vi "num_used_size.vi"(8 "error in (no error)":errorcluster, 11 "worksheet_Refnum":refnum<k7>) -> (0 "error out":errorcluster, 1 "Rows(0)":i32, 2 "Columns(0)":i32, 3 "worksheet_Refnum":refnum<k7>)   [LabVIEW 2015, in "Excel.lvclass"]
uses:
  Excel.lvclass
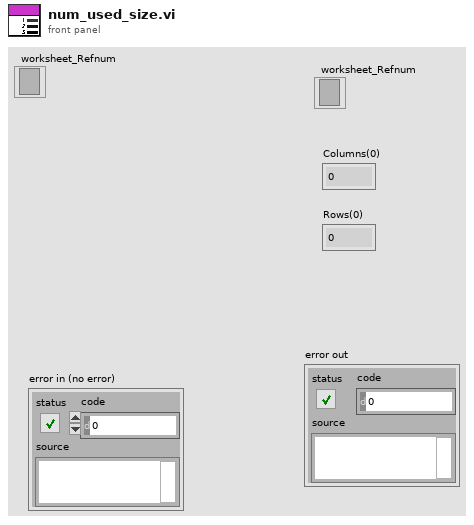
[diagram p1: front panel]
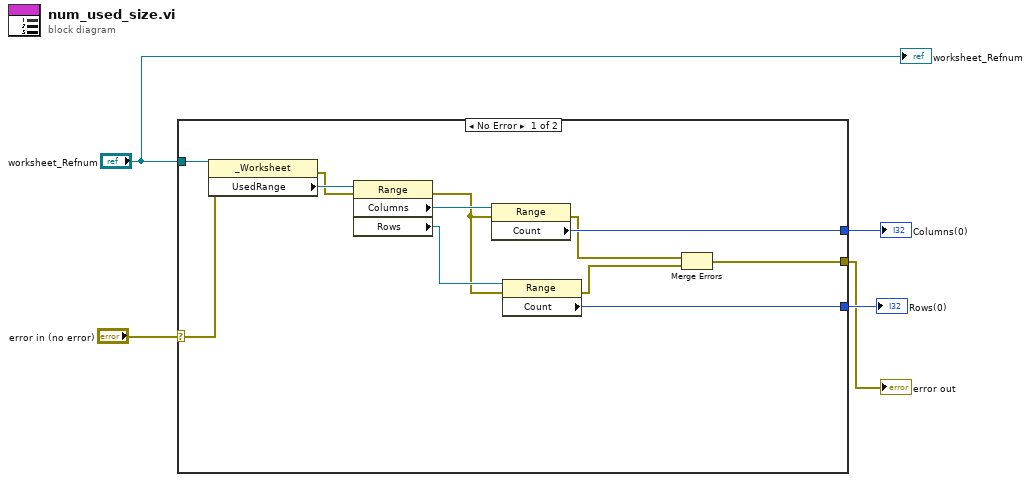
[diagram p0: block diagram]
diagram:
  n1 = case shown="No Error" "error in (no error)" {
    selector: "error in (no error)" -> [w12 w18]
    tunnel: [w16 _] -> w5
    tunnel: [w13 _] -> w4
    tunnel: [w7 w18] -> w2
    tunnel: "worksheet_Refnum" -> [w6 _]
    frame No Error {
      n2 = property class="_Worksheet"(reference=w6, error in=w12) -> (error out=w11:errorcluster, "UsedRange"=w14:refnum<k7>)  [unwired: 1 out]
      n3 = property class="Range"(reference=w14, error in=w11) -> (error out=w10:errorcluster, "Columns"=w15:refnum<k7>, "Rows"=w17:refnum<k7>)  [unwired: 1 out]
      n4 = property class="Range"(reference=w15, error in=w10) -> (error out=w9:errorcluster, "Count"=w13:i32)  [unwired: 1 out]
      n5 = property class="Range"(reference=w17, error in=w10) -> (error out=w8:errorcluster, "Count"=w16:i32)  [unwired: 1 out]
      n6 = Merge Errors(w9, w8) -> (w7:errorcluster)
    }
    frame Error {
    }
  }
  "Columns(0)" <- w4
  "Rows(0)" <- w5
  "error out" <- w2
  "worksheet_Refnum" <- "worksheet_Refnum"
